vi "Scan Code 2 MIDI.vi"(4 "ScanCode":i16) -> (1 "MIDI note":i32)   [LabVIEW 2016]
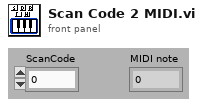
[diagram p1: front panel]
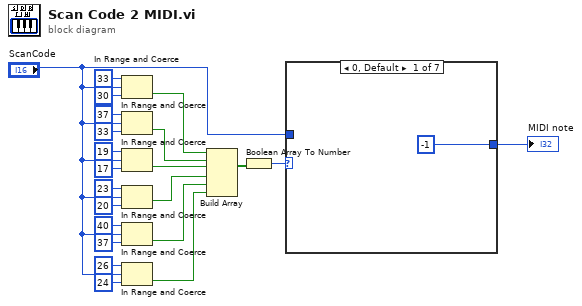
[diagram p0: block diagram]
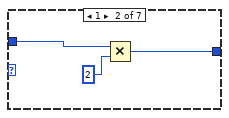
[diagram p2: hidden frame]
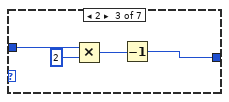
[diagram p3: hidden frame]
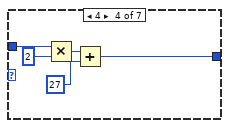
[diagram p4: hidden frame]
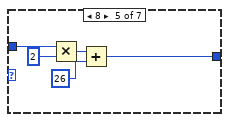
[diagram p5: hidden frame]
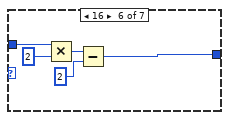
[diagram p6: hidden frame]
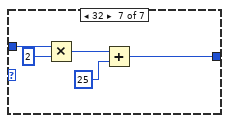
[diagram p7: hidden frame]
diagram:
  n1 = In Range and Coerce(upper limit=i16 33, x="ScanCode", lower limit=i16 30) -> (In Range?=w8:bool)  [unwired: 1 out]
  n2 = In Range and Coerce(upper limit=i16 37, x="ScanCode", lower limit=i16 33) -> (In Range?=w17:bool)  [unwired: 1 out]
  n3 = In Range and Coerce(upper limit=i16 19, x="ScanCode", lower limit=i16 17) -> (In Range?=w9:bool)  [unwired: 1 out]
  n4 = In Range and Coerce(upper limit=i16 23, x="ScanCode", lower limit=i16 20) -> (In Range?=w10:bool)  [unwired: 1 out]
  n5 = In Range and Coerce(upper limit=i16 40, x="ScanCode", lower limit=i16 37) -> (In Range?=w16:bool)  [unwired: 1 out]
  n6 = In Range and Coerce(upper limit=i16 26, x="ScanCode", lower limit=i16 24) -> (In Range?=w22:bool)  [unwired: 1 out]
  n7 = Build Array(w8, w17, w9, w10, w16, w22) -> (w11:bool[])
  n8 = Boolean Array To Number(Boolean array=w11) -> (number=w13:u32)
  n9 = case shown="0, Default" w13 {
    tunnel: "ScanCode" -> [_ w26 w30 w35 w40 w45 w50]
    tunnel: [-1 w24 w27 w31 w36 w41 w46] -> w1
    frame 0, Default {
    }
    frame 1 {
      n10 = Multiply(x=w26, y=i16 2) -> (x*y=w24:i16)
    }
    frame 2 {
      n11 = Multiply(x=w30, y=i16 2) -> (x*y=w28:i16)
      n12 = Decrement(x=w28) -> (x-1=w27:i16)
    }
    frame 4 {
      n13 = Multiply(x=w35, y=i16 2) -> (x*y=w33:i16)
      n14 = Add(x=w33, y=i16 27) -> (x+y=w31:i16)
    }
    frame 8 {
      n15 = Multiply(x=w40, y=i16 2) -> (x*y=w38:i16)
      n16 = Add(x=w38, y=i16 26) -> (x+y=w36:i16)
    }
    frame 16 {
      n17 = Multiply(x=w45, y=i16 2) -> (x*y=w43:i16)
      n18 = Subtract(x=w43, y=i16 2) -> (x-y=w41:i16)
    }
    frame 32 {
      n19 = Multiply(x=w50, y=i16 2) -> (x*y=w48:i16)
      n20 = Add(x=w48, y=i16 25) -> (x+y=w46:i16)
    }
  }
  "MIDI note" <- w1
